vi "wrap_text_in_listbox_column.vi"(7 "width (autosize)":u32, 8 "error_in":errorcluster, 10 "colum_to_wrap":i32, 11 "multicolumn_listbox_reference":refnum<vi>) -> (0 "error_out":errorcluster, 3 "wrapped_lines_count":i32)   [LabVIEW 2020]
doc: "This VI uses the <B>Get Nth Line</B> property to wrap text.\n\nDoug Norman"
uses:
  <vilib>/Utility/miscctls.llb/LVRowAndColumnTypeDef.ctl
panel:
  out "tmp_width_control":string
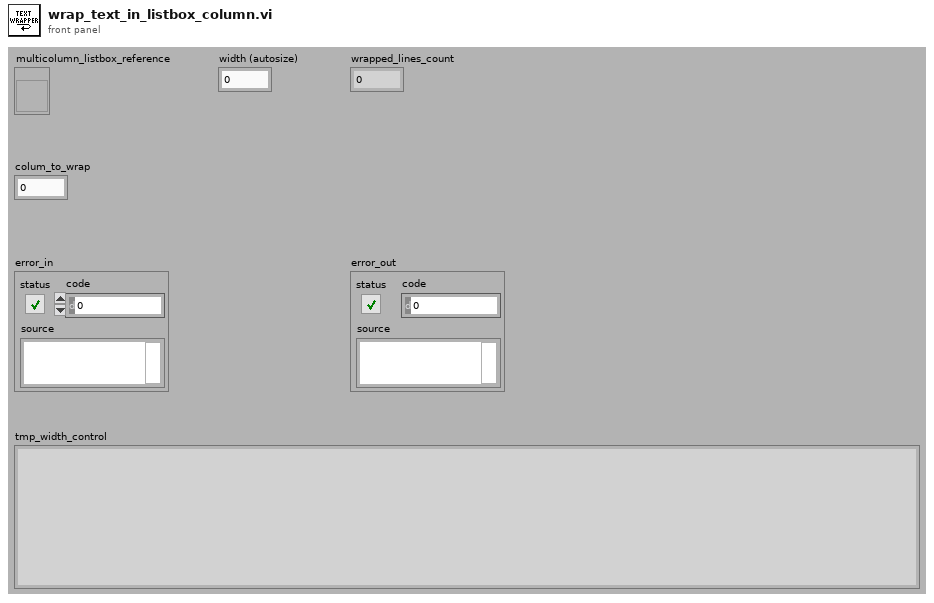
[diagram p1: front panel]
types:
  T1 = typedef "LVRowAndColumnTypeDef.ctl" = cluster{"Row":i32, "Column":i32}
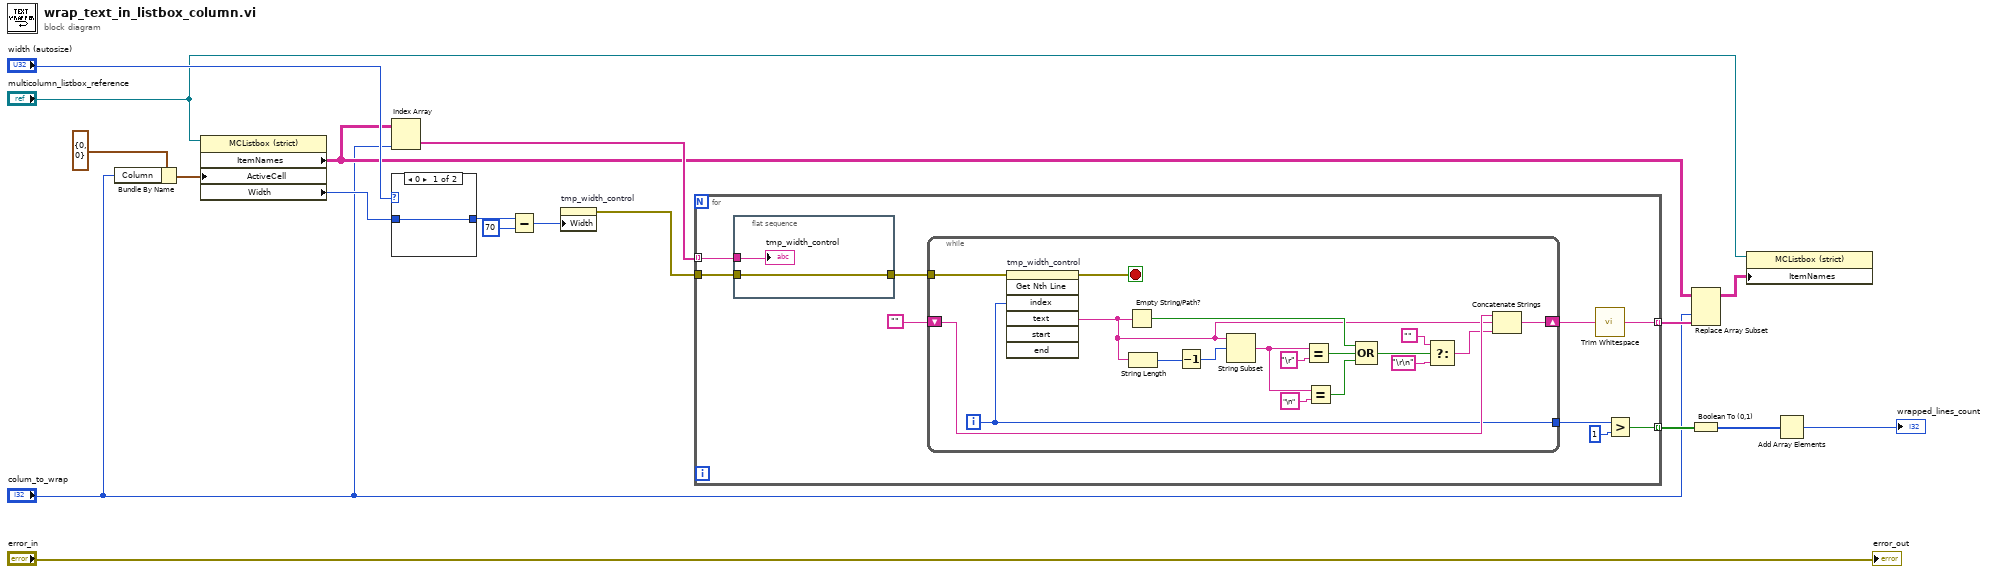
[diagram p0: block diagram]
diagram:
  n1 = Bundle By Name(cluster=T1 {"Row"=0, "Column"=0} ("Active Cell:Active Cell"), "Column"="colum_to_wrap") -> (w11:T1)
  n2 = property class="MCListbox (strict)"(reference="multicolumn_listbox_reference", "ActiveCell"=w11) -> ("ItemNames"=w8:string[][], "Width"=w13:u32)  [unwired: 1 in, 2 out]
  n3 = Index Array(array=w8, index (col)="colum_to_wrap") -> (element=w15:string[])  [unwired: 1 in]
  n4 = case shown="0" "width (autosize)" {
    selector: "width (autosize)" -> [_ w20]
    tunnel: w13 -> [w19 _]
    tunnel: [w19 w20] -> w3
    frame 0 {
    }
    frame Default {
    }
  }
  n5 = Subtract(x=w3, y=u32 70) -> (x-y=w2:u32)
  n6 = property on="tmp_width_control" class="Str"("Width"=w2) -> (error out=w10:errorcluster)  [unwired: 2 in, 1 out]
  n7 = for {
    tunnel: [w29] -> w7 mode=indexing
    tunnel: [w28] -> w18 mode=indexing
    tunnel: w15 -> [w27] mode=indexing
    tunnel: w10 -> [w22]
    n8 = flat-sequence {
      tunnel: w27 -> [w31]
      tunnel: w22 -> [w30]
      tunnel: [w30] -> w21
      frame #0 {
        "tmp_width_control" <- w31
      }
    }
    n9 = while {
      shift-right: [w46] -> w25
      shift-left: "" -> [w49]
      tunnel: [w45] -> w24
      tunnel: w21 -> [w33]
      i -> [w45]
      stop <- w32 stop-if-true
      n10 = invoke on="tmp_width_control" class="Str" method="Get Nth Line"(error in=w33, "index"=w45) -> (error out=w32:errorcluster, "text"=w38:string)  [unwired: 5 in, 5 out]
      n11 = Empty String/Path?(string/path=w38) -> (empty?=w42:bool)
      n12 = String Length(string=w38) -> (length=w43:i32)
      n13 = Decrement(x=w43) -> (x-1=w37:i32)
      n14 = String Subset(string=w38, offset (0)=w37) -> (substring=w36:string)  [unwired: 1 in]
      n15 = Equal?(x=w36, y="\r") -> (x = y?=w41:bool)
      n16 = Equal?(x=w36, y="\n") -> (x = y?=w40:bool)
      n17 = Compound Arithmetic op=OR(w42, w41, w40) -> (w39:bool)
      n18 = Select(t="", s=w39, f="\r\n") -> (s? t:f=w47:string)
      n19 = Concatenate Strings(w49, w38, w47) -> (w46:string)
    }
    n20 = call <vilib>:"Trim Whitespace.vi"("string"=w25) -> ("trimmed string"=w29:string)  [unwired: 1 in]
    n21 = Greater?(x=w24, y=1) -> (0:w28:bool)
  }
  n22 = Boolean To (0,1)(Boolean=w18) -> (0, 1=w17:i16[])
  n23 = Replace Array Subset(array=w8, new element=w7, index (col)="colum_to_wrap") -> (w5:string[][])  [unwired: 1 in]
  n24 = property class="MCListbox (strict)"(reference="multicolumn_listbox_reference", "ItemNames"=w5) -> ()  [unwired: 1 in, 2 out]
  n25 = Add Array Elements(numeric array=w17) -> (sum=→"wrapped_lines_count":i16)
  "error_out" <- "error_in"
